vi "Acc2LabVIEWData_Float64.vi"(1 "Acc_Data_In":T1[](array[typedef]), 5 "error in":errorcluster) -> (15 "Acc_Data_Out":T1[](array[typedef]), 17 "Value":dbl, 19 "error out":errorcluster)   [LabVIEW 2014, in "ACC_LabVIEW.lvlib"]
uses:
  ACC_LabVIEW.lvlib
  ACC_LabVIEW_Container.ctl
  ACC_LabVIEW_DataTypes.ctl
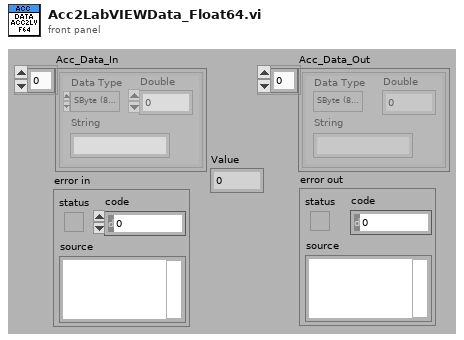
[diagram p1: front panel]
types:
  T1 = typedef "ACC_LabVIEW.lvlib/ACC_LabVIEW_Container.ctl" = cluster{"Data Type":T2, "String":string, "Double":dbl}
  T2 = typedef "ACC_LabVIEW.lvlib/ACC_LabVIEW_DataTypes.ctl" = enum16{"SByte (8Bit Int signed)", "UByte (8Bit int unsigned)", "SWord (16Bit Int signed)", "UWord (16Bit Int unsigned)", "SLong (32Bit Int signed)", "ULong (32Bit Int unsigned)", "Float32 (float)", "Float64 (double)", "String"}
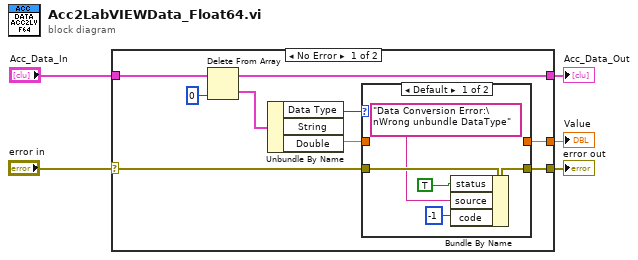
[diagram p0: block diagram]
diagram:
  n1 = case shown="No Error" "error in" {
    selector: "error in" -> [w8 w23]
    tunnel: "Acc_Data_In" -> [w14 w22]
    tunnel: [w13 w22] -> w4
    tunnel: [w7 w23] -> w2
    tunnel: [w6 _] -> w1
    frame No Error {
      n2 = Delete From Array(array=w14, index=0) -> (deleted portion=w12:T1, array with subset deleted=w13:T1[])  [unwired: 1 in]
      n3 = Unbundle By Name(w12) -> ("Data Type"=w11:T2, "Double"=w10:dbl)  [unwired: 1 out]
      n4 = case shown="Default" w11 {
        tunnel: w10 -> [_ w21]
        tunnel: [_ w21] -> w6
        tunnel: w8 -> [w19 w20]
        tunnel: [w18 w20] -> w7
        frame Default {
          n5 = Bundle By Name(cluster=w19, "status"=TRUE, "source"="Data Conversion Error:\nWrong unbundle DataType", "code"=-1) -> (w18:errorcluster)
        }
        frame "Float64 (double)" {
        }
      }
    }
    frame Error {
    }
  }
  "Acc_Data_Out" <- w4
  "error out" <- w2
  "Value" <- w1
